vi "tp4-1-bis.vi"() -> ()   [LabVIEW 2013]
uses:
  <vilib>/gmath/statdist.llb/Normal Inverse CDF.vi
  <vilib>/gmath/NI_Gmath.lvlib
panel:
  out "P":i32
  in  "Vector":i64
  in  "Cancel Button":bool
  out "Waveform Chart":cluster{"x":dbl, dbl}(graph)
  in  "Nivel de Ruido":dbl=30.0
  in  "Medicion":dbl
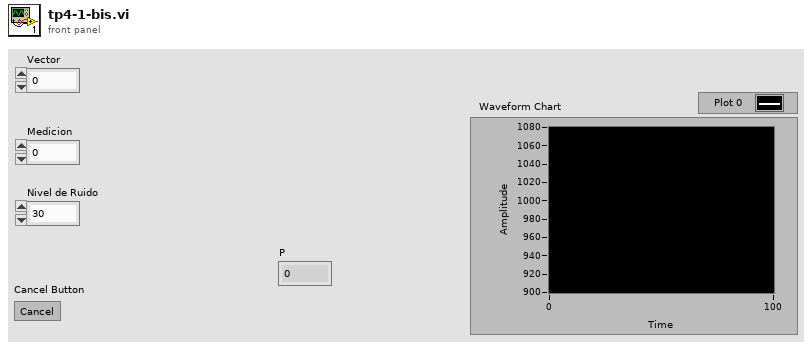
[diagram p1: front panel]
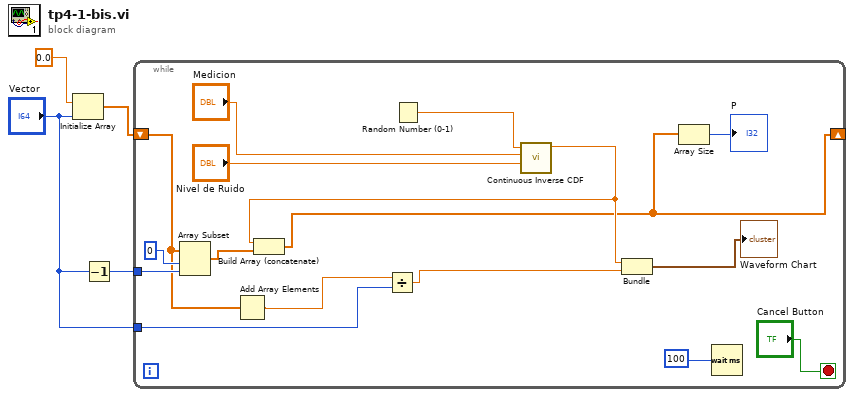
[diagram p0: block diagram]
diagram:
  n1 = Initialize Array(0.0, "Vector") -> (w2:dbl[])
  n2 = Decrement(x="Vector") -> (x-1=w3:i64)
  n3 = while {
    tunnel: w3 -> [w12]
    shift-right: [w6] -> _
    shift-left: w2 -> [w8]
    tunnel: "Vector" -> [w7]
    stop <- "Cancel Button" stop-if-true
    n4 = Array Subset(array=w8, index=0, length=w12) -> (w10:dbl[])
    n5 = Add Array Elements(numeric array=w8) -> (sum=w13:dbl)
    n6 = Divide(x=w13, y=w7) -> (x/y=w16:dbl)
    n7 = Random Number (0-1)() -> (number: 0 to 1=w17:dbl)
    n8 = call-poly <vilib>:"Continuous Inverse CDF.vi"("std"="Nivel de Ruido", "mean"="Medicion", "cdf(x)"=w17) -> ("x"=w9:dbl)  [unwired: 7 in, 1 out]
    n9 = Build Array (concatenate)(w9, w10) -> (w6:dbl[])
    n10 = Bundle("x"=w9, w16) -> (→"Waveform Chart":cluster{"x":dbl, dbl})  [unwired: 1 in]
    n11 = Array Size(array=w6) -> (size(s)=→"P":i32)
    n12 = Wait (ms)(milliseconds to wait=100) -> ()  [unwired: 1 out]
  }
